vi "NI-DCPower Source DC Current.vi"() -> ()   [LabVIEW 2021]
doc: "Demonstrates how to use the DC Current Output Function to force an output current. This example initializes a session, configures the Output Function, Sense, Autorange, Current Level and Voltage Limit, initiates generation, waits for a specified delay, and measures the voltage and current output. This example uses Single Point source mode."
uses:
  <instrlib>/niDCPower/nidcpower.llb/niDCPower Source Mode.ctl
  <instrlib>/niDCPower/nidcpower.llb/niDCPower Wait For Event - Event.ctl
  <instrlib>/niDCPower/nidcpower.llb/niDCPower Output Function.ctl
panel:
  in  "error in":errorcluster
  out "error out":errorcluster
  in  "Source Delay (Sec)":dbl=0.1 format="%.3p"
  out "Voltage Measurement":dbl
  out "Current Measurement":dbl
  in  "Voltage Limit Range":dbl=6.0 format="%.5p"
  in  "Current Level Range":dbl=0.01 format="%.3p"
  in  "Voltage Limit":dbl=2.0 format="%.5p"
  in  "Current Level":dbl=0.01 format="%.3p"
  in  "Load SMU Channel":string="0"
  in  "Load SMU":refnum<k15>="Dev1"
  # "Overview: Demonstrates how to use the DC Current Output Function to force an output current.  \nThis example initializes a session; configures the Output Function, Current Level and Voltage Limit; \ninitiates generation; waits for a specified delay; and measures the voltage and current output.  \nRequirements: NI-DCPower\nInstructions:\n1. Select the appropriate device in the Resource Name control.\n2. Configure the parameters of the DC Current signal you'd like to output.\n3. Run the VI."
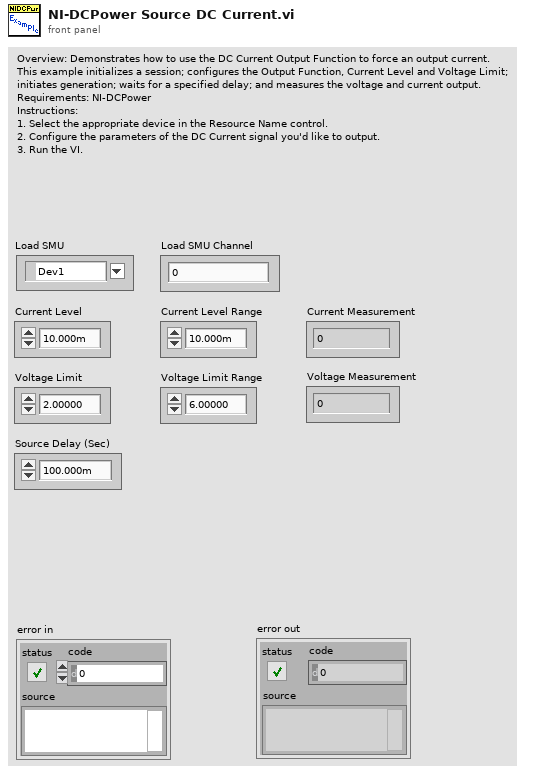
[diagram p1: front panel]
types:
  T1 = typedef "niDCPower Output Function.ctl" = i32
  T2 = typedef "niDCPower Wait For Event - Event.ctl" = i32
  T3 = typedef "niDCPower Source Mode.ctl" = i32
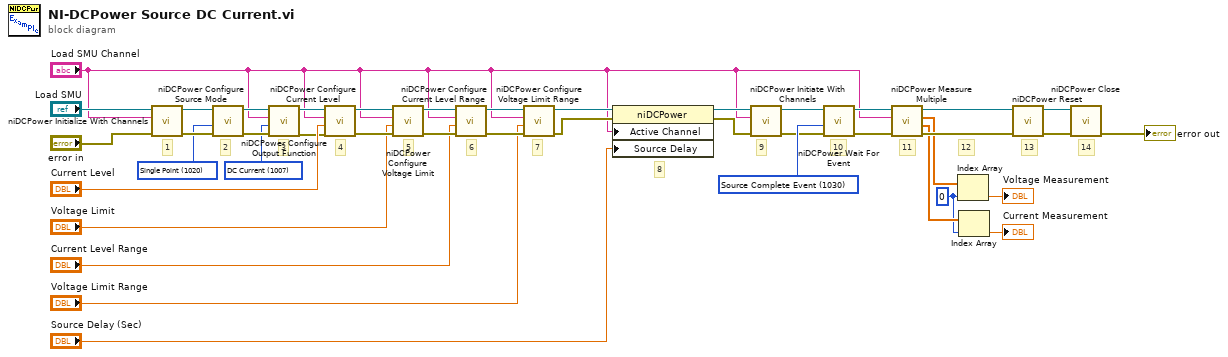
[diagram p0: block diagram]
diagram:
  w8 = T1 1007 items=["DC Voltage"=1006, "DC Current"=1007, "Pulse Voltage"=1049, "Pulse Current"=1050] ("output function")
  w11 = T2 1030 items=["Source Complete Event"=1030, "Measure Complete Event"=1031, "Sequence Iteration Complete Event"=1032, "Sequence Engine Done Event"=1033] ("event")
  w19 = 0 ("index")
  w30 = T3 1020 items=["Single Point"=1020, "Sequence"=1021] ("source mode")
  # "14"
  # "8"
  # "11"
  # "10"
  # "7"
  # "6"
  # "2"
  # "3"
  # "12"
  # "13"
  # "9"
  # "5"
  # "4"
  # "1"
  n1 = call <instrlib>:"niDCPower Initialize With Channels.vi"("error in (no error)"="error in", "channels"="Load SMU Channel", "resource name"="Load SMU") -> ("error out"=w34:errorcluster, "instrument handle out"=w33:refnum<k15>)  [unwired: 2 in, 5 out]
  n2 = call <instrlib>:"niDCPower Configure Source Mode.vi"("error in (no error)"=w34, "source mode"=w30, "instrument handle"=w33) -> ("error out"=w32:errorcluster, "instrument handle out"=w31:refnum<k15>)  [unwired: 7 out]
  n3 = call <instrlib>:"niDCPower Configure Output Function.vi"("error in (no error)"=w32, "output function"=w8, "channel name"="Load SMU Channel", "instrument handle"=w31) -> ("error out"=w10:errorcluster, "instrument handle out"=w9:refnum<k15>)  [unwired: 6 out]
  n4 = call <instrlib>:"niDCPower Configure Current Level.vi"("error in (no error)"=w10, "current level"="Current Level", "channel name"="Load SMU Channel", "instrument handle"=w9) -> ("error out"=w39:errorcluster, "instrument handle out"=w40:refnum<k15>)  [unwired: 6 out]
  n5 = call <instrlib>:"niDCPower Configure Voltage Limit.vi"("error in (no error)"=w39, "voltage limit"="Voltage Limit", "channel name"="Load SMU Channel", "instrument handle"=w40) -> ("error out"=w29:errorcluster, "instrument handle out"=w28:refnum<k15>)  [unwired: 6 out]
  n6 = call <instrlib>:"niDCPower Configure Current Level Range.vi"("error in (no error)"=w29, "current level range"="Current Level Range", "channel name"="Load SMU Channel", "instrument handle"=w28) -> ("error out"=w27:errorcluster, "instrument handle out"=w26:refnum<k15>)  [unwired: 6 out]
  n7 = call <instrlib>:"niDCPower Configure Voltage Limit Range.vi"("error in (no error)"=w27, "voltage limit range"="Voltage Limit Range", "channel name"="Load SMU Channel", "instrument handle"=w26) -> ("error out"=w15:errorcluster, "instrument handle out"=w16:refnum<k15>)  [unwired: 6 out]
  n8 = property class="niDCPower"(reference=w16, error in=w15, "Active Channel"="Load SMU Channel", "Source Delay"="Source Delay (Sec)") -> (reference out=w5:refnum<k15>, error out=w2:errorcluster)
  n9 = call <instrlib>:"niDCPower Initiate With Channels.vi"("error in (no error)"=w2, "channel name"="Load SMU Channel", "instrument handle"=w5) -> ("error out"=w4:errorcluster, "instrument handle out"=w3:refnum<k15>)  [unwired: 7 in]
  n10 = call <instrlib>:"niDCPower Wait For Event.vi"("error in (no error)"=w4, "event"=w11, "instrument handle"=w3) -> ("error out"=w12:errorcluster, "instrument handle out"=w13:refnum<k15>)  [unwired: 1 in, 6 out]
  n11 = call <instrlib>:"niDCPower Measure Multiple.vi"("error in (no error)"=w12, "channel name"="Load SMU Channel", "instrument handle"=w13) -> ("error out"=w22:errorcluster, "current measurements"=w20:dbl[], "voltage measurements"=w21:dbl[], "instrument handle out"=w23:refnum<k15>)  [unwired: 5 out]
  n12 = Index Array(array=w21, index=w19) -> (element=→"Voltage Measurement":dbl)
  n13 = Index Array(array=w20, index=w19) -> (element=→"Current Measurement":dbl)
  n14 = call <instrlib>:"niDCPower Reset.vi"("error in (no error)"=w22, "instrument handle"=w23) -> ("error out"=w36:errorcluster, "instrument handle out"=w37:refnum<k15>)  [unwired: 2 in, 6 out]
  n15 = call <instrlib>:"niDCPower Close.vi"("error in (no error)"=w36, "instrument handle"=w37) -> ("error out"=→"error out":errorcluster)  [unwired: 9 out]
